vi "Methods to Method Info.vi"(10 "Class":string, 11 "Methods from Node":T2(array[cluster])) -> (2 "Methods for Tree":T1(array[cluster]), 3 "Methods[]":T3(array[cluster]))   [LabVIEW 2023] (continued)
From Typedefs"}, "Method Flags"={"IsDeprecated"=FALSE, "IsPrivate"=FALSE, "IsScripting"=FALSE, "IsNotInRun-Time"=FALSE}, "Divider"=FALSE}, {"Class Info"={"Unique ID string"="82", "Parent ID string"="", "Class Name (unlocalized)"="TagSet", "Class Name (localized)"="TagSet"}, "Method Info"={"Unique ID string"="5d1e4400", "Data name"="Get", "Short name (localized)"="Get", "Long name (localized)"="Get"}, "Method Flags"={"IsDeprecated"=FALSE, "IsPrivate"=TRUE, "IsScripting"=FALSE, "IsNotInRun-Time"=TRUE}, "Divider"=FALSE}, {"Class Info"={"Unique ID string"="82", "Parent ID string"="", "Class Name (unlocalized)"="TagSet", "Class Name (localized)"="TagSet"}, "Method Info"={"Unique ID string"="5d1e4401", "Data name"="Set", "Short name (localized)"="Set", "Long name (localized)"="Set"}, "Method Flags"={"IsDeprecated"=FALSE, "IsPrivate"=TRUE, "IsScripting"=FALSE, "IsNotInRun-Time"=TRUE}, "Divider"=FALSE}, {"Class Info"={"Unique ID string"="82", "Parent ID string"="", "Class Name (unlocalized)"="TagSet", "Class Name (localized)"="TagSet"}, "Method Info"={"Unique ID string"="5d1e4402", "Data name"="Set XML", "Short name (localized)"="Set XML", "Long name (localized)"="Set XML"}, "Method Flags"={"IsDeprecated"=FALSE, "IsPrivate"=TRUE, "IsScripting"=FALSE, "IsNotInRun-Time"=TRUE}, "Divider"=FALSE}, {"Class Info"={"Unique ID string"="82", "Parent ID string"="", "Class Name (unlocalized)"="TagSet", "Class Name (localized)"="TagSet"}, "Method Info"={"Unique ID string"="5d1e4403", "Data name"="Get XML", "Short name (localized)"="Get XML", "Long name (localized)"="Get XML"}, "Method Flags"={"IsDeprecated"=FALSE, "IsPrivate"=TRUE, "IsScripting"=FALSE, "IsNotInRun-Time"=TRUE}, "Divider"=FALSE}, {"Class Info"={"Unique ID string"="84", "Parent ID string"="123", "Class Name (unlocalized)"="SceneWindow", "Class Name (localized)"="SceneWindow"}, "Method Info"={"Unique ID string"="c55e400", "Data name"="Setup Camera", "Short name (localized)"="Setup Camera", "Long name (localized)"="Setup Camera"}, "Method Flags"={"IsDeprecated"=FALSE, "IsPrivate"=FALSE, "IsScripting"=FALSE, "IsNotInRun-Time"=FALSE}, "Divider"=FALSE}, {"Class Info"={"Unique ID string"="84", "Parent ID string"="123", "Class Name (unlocalized)"="SceneWindow", "Class Name (localized)"="SceneWindow"}, "Method Info"={"Unique ID string"="c55e401", "Data name"="Projection.Frustum", "Short name (localized)"="Projection.Frustum", "Long name (localized)"="Projection:Frustum"}, "Method Flags"={"IsDeprecated"=FALSE, "IsPrivate"=FALSE, "IsScripting"=FALSE, "IsNotInRun-Time"=FALSE}, "Divider"=FALSE}, {"Class Info"={"Unique ID string"="84", "Parent ID string"="123", "Class Name (unlocalized)"="SceneWindow", "Class Name (localized)"="SceneWindow"}, "Method Info"={"Unique ID string"="c55e402", "Data name"="Projection.Orthographic", "Short name (localized)"="Projection.Orthographic", "Long name (localized)"="Projection:Orthographic"}, "Method Flags"={"IsDeprecated"=FALSE, "IsPrivate"=FALSE, "IsScripting"=FALSE, "IsNotInRun-Time"=FALSE}, "Divider"=FALSE}, {"Class Info"={"Unique ID string"="84", "Parent ID string"="123", "Class Name (unlocalized)"="SceneWindow", "Class Name (localized)"="SceneWindow"}, "Method Info"={"Unique ID string"="c55e403", "Data name"="Projection.Perspective", "Short name (localized)"="Projection.Perspective", "Long name (localized)"="Projection:Perspective"}, "Method Flags"={"IsDeprecated"=FALSE, "IsPrivate"=FALSE, "IsScripting"=FALSE, "IsNotInRun-Time"=FALSE}, "Divider"=FALSE}, {"Class Info"={"Unique ID string"="84", "Parent ID string"="123", "Class Name (unlocalized)"="SceneWindow", "Class Name (localized)"="SceneWindow"}, "Method Info"={"Unique ID string"="c55e404", "Data name"="Render to Image", "Short name (localized)"="Render to Image", "Long name (localized)"="Render to Image"}, "Method Flags"={"IsDeprecated"=FALSE, "IsPrivate"=FALSE, "IsScripting"=FALSE, "IsNotInRun-Time"=FALSE}, "Divider"=FALSE}, {"Class Info"={"Unique ID string"="84", "Parent ID string"="123", "Class Name (unlocalized)"="SceneWindow", "Class Name (localized)"="SceneWindow"}, "Method Info"={"Unique ID string"="c55e405", "Data name"="Pick", "Short name (localized)"="Pick", "Long name (localized)"="Pick"}, "Method Flags"={"IsDeprecated"=FALSE, "IsPrivate"=FALSE, "IsScripting"=FALSE, "IsNotInRun-Time"=FALSE}, "Divider"=FALSE}, {"Class Info"={"Unique ID string"="84", "Parent ID string"="123", "Class Name (unlocalized)"="SceneWindow", "Class Name (localized)"="SceneWindow"}, "Method Info"={"Unique ID string"="c55e406", "Data name"="Redraw", "Short name (localized)"="Redraw", "Long name (localized)"="Redraw"}, "Method Flags"={"IsDeprecated"=FALSE, "IsPrivate"=FALSE, "IsScripting"=FALSE, "IsNotInRun-Time"=FALSE}, "Divider"=FALSE}, {"Class Info"={"Unique ID string"="84", "Parent ID string"="123", "Class Name (unlocalized)"="SceneWindow", "Class Name (localized)"="SceneWindow"}, "Method Info"={"Unique ID string"="c55e407", "Data name"="AutoFocus", "Short name (localized)"="AutoFocus", "Long name (localized)"="AutoFocus"}, "Method Flags"={"IsDeprecated"=FALSE, "IsPrivate"=FALSE, "IsScripting"=FALSE, "IsNotInRun-Time"=FALSE}, "Divider"=FALSE}, {"Class Info"={"Unique ID string"="84", "Parent ID string"="123", "Class Name (unlocalized)"="SceneWindow", "Class Name (localized)"="SceneWindow"}, "Method Info"={"Unique ID string"="c55e408", "Data name"="WindowToObjectCoords", "Short name (localized)"="WindowToObjectCoords", "Long name (localized)"="WindowToObjectCoords"}, "Method Flags"={"IsDeprecated"=FALSE, "IsPrivate"=FALSE, "IsScripting"=FALSE, "IsNotInRun-Time"=FALSE}, "Divider"=FALSE}, {"Class Info"={"Unique ID string"="85", "Parent ID string"="80", "Class Name (unlocalized)"="LVClassLibrary", "Class Name (localized)"="LVClassLibrary"}, "Method Info"={"Unique ID string"="97d6c01", "Data name"="Add Property", "Short name (localized)"="Add Property", "Long name (localized)"="Add Property"}, "Method Flags"={"IsDeprecated"=FALSE, "IsPrivate"=TRUE, "IsScripting"=TRUE, "IsNotInRun-Time"=FALSE}, "Divider"=FALSE}, {"Class Info"={"Unique ID string"="85", "Parent ID string"="80", "Class Name (unlocalized)"="LVClassLibrary", "Class Name (localized)"="LVClassLibrary"}, "Method Info"={"Unique ID string"="97d6c02", "Data name"="Add Dynamic Member VI", "Short name (localized)"="Add Dynamic Member VI", "Long name (localized)"="Add Dynamic Member VI"}, "Method Flags"={"IsDeprecated"=FALSE, "IsPrivate"=TRUE, "IsScripting"=TRUE, "IsNotInRun-Time"=FALSE}, "Divider"=FALSE}, {"Class Info"={"Unique ID string"="85", "Parent ID string"="80", "Class Name (unlocalized)"="LVClassLibrary", "Class Name (localized)"="LVClassLibrary"}, "Method Info"={"Unique ID string"="97d6c03", "Data name"="Add Static Member VI", "Short name (localized)"="Add Static Member VI", "Long name (localized)"="Add Static Member VI"}, "Method Flags"={"IsDeprecated"=FALSE, "IsPrivate"=TRUE, "IsScripting"=TRUE, "IsNotInRun-Time"=FALSE}, "Divider"=FALSE}, {"Class Info"={"Unique ID string"="85", "Parent ID string"="80", "Class Name (unlocalized)"="LVClassLibrary", "Class Name (localized)"="LVClassLibrary"}, "Method Info"={"Unique ID string"="97d6c04", "Data name"="Add Probe", "Short name (localized)"="Add Probe", "Long name (localized)"="Add Probe"}, "Method Flags"={"IsDeprecated"=FALSE, "IsPrivate"=TRUE, "IsScripting"=TRUE, "IsNotInRun-Time"=FALSE}, "Divider"=FALSE}, {"Class Info"={"Unique ID string"="85", "Parent ID string"="80", "Class Name (unlocalized)"="LVClassLibrary", "Class Name (localized)"="LVClassLibrary"}, "Method Info"={"Unique ID string"="97d6c05", "Data name"="Remove Property", "Short name (localized)"="Remove Property", "Long name (localized)"="Remove Property"}, "Method Flags"={"IsDeprecated"=FALSE, "IsPrivate"=TRUE, "IsScripting"=TRUE, "IsNotInRun-Time"=FALSE}, "Divider"=FALSE}, {"Class Info"={"Unique ID string"="85", "Parent ID string"="80", "Class Name (unlocalized)"="LVClassLibrary", "Class Name (localized)"="LVClassLibrary"}, "Method Info"={"Unique ID string"="97d6c06", "Data name"="Remove Member VI", "Short name (localized)"="Remove Member VI", "Long name (localized)"="Remove Member VI"}, "Method Flags"={"IsDeprecated"=FALSE, "IsPrivate"=TRUE, "IsScripting"=TRUE, "IsNotInRun-Time"=FALSE}, "Divider"=FALSE}, {"Class Info"={"Unique ID string"="85", "Parent ID string"="80", "Class Name (unlocalized)"="LVClassLibrary", "Class Name (localized)"="LVClassLibrary"}, "Method Info"={"Unique ID string"="97d6c07", "Data name"="Remove Probe", "Short name (localized)"="Remove Probe", "Long name (localized)"="Remove Probe"}, "Method Flags"={"IsDeprecated"=FALSE, "IsPrivate"=TRUE, "IsScripting"=TRUE, "IsNotInRun-Time"=FALSE}, "Divider"=FALSE}, {"Class Info"={"Unique ID string"="85", "Parent ID string"="80", "Class Name (unlocalized)"="LVClassLibrary", "Class Name (localized)"="LVClassLibrary"}, "Method Info"={"Unique ID string"="97d6c09", "Data name"="Clone Member Data", "Short name (localized)"="Clone Member Data", "Long name (localized)"="Clone Member Data"}, "Method Flags"={"IsDeprecated"=FALSE, "IsPrivate"=TRUE, "IsScripting"=TRUE, "IsNotInRun-Time"=FALSE}, "Divider"=FALSE}, {"Class Info"={"Unique ID string"="85", "Parent ID string"="80", "Class Name (unlocalized)"="LVClassLibrary", "Class Name (localized)"="LVClassLibrary"}, "Method Info"={"Unique ID string"="97d6c0a", "Data name"="Set Member Data", "Short name (localized)"="Set Member Data", "Long name (localized)"="Set Member Data"}, "Method Flags"={"IsDeprecated"=FALSE, "IsPrivate"=TRUE, "IsScripting"=TRUE, "IsNotInRun-Time"=FALSE}, "Divider"=FALSE}, {"Class Info"={"Unique ID string"="85", "Parent ID string"="80", "Class Name (unlocalized)"="LVClassLibrary", "Class Name (localized)"="LVClassLibrary"}, "Method Info"={"Unique ID string"="97d6c0b", "Data name"="Get MustOverride?", "Short name (localized)"="Get MustOverride?", "Long name (localized)"="Descendants Must Override Item?:Get"}, "Method Flags"={"IsDeprecated"=FALSE, "IsPrivate"=FALSE, "IsScripting"=FALSE, "IsNotInRun-Time"=TRUE}, "Divider"=FALSE}, {"Class Info"={"Unique ID string"="85", "Parent ID string"="80", "Class Name (unlocalized)"="LVClassLibrary", "Class Name (localized)"="LVClassLibrary"}, "Method Info"={"Unique ID string"="97d6c0c", "Data name"="Set MustOverride?", "Short name (localized)"="Set MustOverride?", "Long name (localized)"="Descendants Must Override Item?:Set"}, "Method Flags"={"IsDeprecated"=FALSE, "IsPrivate"=FALSE, "IsScripting"=FALSE, "IsNotInRun-Time"=TRUE}, "Divider"=FALSE}, {"Class Info"={"Unique ID string"="85", "Parent ID string"="80", "Class Name (unlocalized)"="LVClassLibrary", "Class Name (localized)"="LVClassLibrary"}, "Method Info"={"Unique ID string"="97d6c0d", "Data name"="Get MustCallParent?", "Short name (localized)"="Get MustCallParent?", "Long name (localized)"="Descendants Must Call Parent Item?:Get"}, "Method Flags"={"IsDeprecated"=FALSE, "IsPrivate"=FALSE, "IsScripting"=FALSE, "IsNotInRun-Time"=TRUE}, "Divider"=FALSE}, {"Class Info"={"Unique ID string"="85", "Parent ID string"="80", "Class Name (unlocalized)"="LVClassLibrary", "Class Name (localized)"="LVClassLibrary"}, "Method Info"={"Unique ID string"="97d6c0e", "Data name"="Set MustCallParent?", "Short name (localized)"="Set MustCallParent?", "Long name (localized)"="Descendants Must Call Parent Item?:Set"}, "Method Flags"={"IsDeprecated"=FALSE, "IsPrivate"=FALSE, "IsScripting"=FALSE, "IsNotInRun-Time"=TRUE}, "Divider"=FALSE}, {"Class Info"={"Unique ID string"="85", "Parent ID string"="80", "Class Name (unlocalized)"="LVClassLibrary", "Class Name (localized)"="LVClassLibrary"}, "Method Info"={"Unique ID string"="97d6c0f", "Data name"="HasImplementation", "Short name (localized)"="HasImplementation", "Long name (localized)"="Has Implementation?"}, "Method Flags"={"IsDeprecated"=FALSE, "IsPrivate"=FALSE, "IsScripting"=FALSE, "IsNotInRun-Time"=TRUE}, "Divider"=FALSE}, {"Class Info"={"Unique ID string"="85", "Parent ID string"="80", "Class Name (unlocalized)"="LVClassLibrary", "Class Name (localized)"="LVClassLibrary"}, "Method Info"={"Unique ID string"="97d6c10", "Data name"="Get Prop Def Folder by Unique ID", "Short name (localized)"="Get Prop Def Folder by Unique ID", "Long name (localized)"="Get Property Definition Folder by Unique ID"}, "Method Flags"={"IsDeprecated"=FALSE, "IsPrivate"=TRUE, "IsScripting"=TRUE, "IsNotInRun-Time"=TRUE}, "Divider"=FALSE}, {"Class Info"={"Unique ID string"="85", "Parent ID string"="80", "Class Name (unlocalized)"="LVClassLibrary", "Class Name (localized)"="LVClassLibrary"}, "Method Info"={"Unique ID string"="97d6c11", "Data name"="DeParent Class", "Short name (localized)"="DeParent Class", "Long name (localized)"="DeParent Class"}, "Method Flags"={"IsDeprecated"=FALSE, "IsPrivate"=TRUE, "IsScripting"=TRUE, "IsNotInRun-Time"=TRUE}, "Divider"=FALSE}, {"Class Info"={"Unique ID string"="87", "Parent ID string"="2", "Class Name (unlocalized)"="MethodVI", "Class Name (localized)"="MethodVI"}, "Method Info"={"Unique ID string"="69a73c00", "Data name"="Invoke Method Editor", "Short name (localized)"="Invoke Method Editor", "Long name (localized)"="Invoke Method Editor"}, "Method Flags"={"IsDeprecated"=FALSE, "IsPrivate"=TRUE, "IsScripting"=FALSE, "IsNotInRun-Time"=FALSE}, "Divider"=FALSE}, {"Class Info"={"Unique ID string"="91", "Parent ID string"="", "Class Name (unlocalized)"="LVTarget", "Class Name (localized)"="LVTarget"}, "Method Info"={"Unique ID string"="5d37bc00", "Data name"="Get Attributes", "Short name (localized)"="Get Attributes", "Long name (localized)"="Get Attributes"}, "Method Flags"={"IsDeprecated"=FALSE, "IsPrivate"=TRUE, "IsScripting"=FALSE, "IsNotInRun-Time"=FALSE}, "Divider"=FALSE}, {"Class Info"={"Unique ID string"="91", "Parent ID string"="", "Class Name (unlocalized)"="LVTarget", "Class Name (localized)"="LVTarget"}, "Method Info"={"Unique ID string"="5d37bc01", "Data name"="Set Attributes", "Short name (localized)"="Set Attributes", "Long name (localized)"="Set Attributes"}, "Method Flags"={"IsDeprecated"=FALSE, "IsPrivate"=TRUE, "IsScripting"=FALSE, "IsNotInRun-Time"=FALSE}, "Divider"=FALSE}, {"Class Info"={"Unique ID string"="91", "Parent ID string"="", "Class Name (unlocalized)"="LVTarget", "Class Name (localized)"="LVTarget"}, "Method Info"={"Unique ID string"="5d37bc02", "Data name"="Custom Command", "Short name (localized)"="Custom Command", "Long name (localized)"="Custom Command"}, "Method Flags"={"IsDeprecated"=FALSE, "IsPrivate"=TRUE, "IsScripting"=FALSE, "IsNotInRun-Time"=FALSE}, "Divider"=FALSE}, {"Class Info"={"Unique ID string"="91", "Parent ID string"="", "Class Name (unlocalized)"="LVTarget", "Class Name (localized)"="LVTarget"}, "Method Info"={"Unique ID string"="5d37c003", "Data name"="LocateFile", "Short name (localized)"="LocateFile", "Long name (localized)"="Locate File or Folder"}, "Method Flags"={"IsDeprecated"=FALSE, "IsPrivate"=TRUE, "IsScripting"=FALSE, "IsNotInRun-Time"=FALSE}, "Divider"=FALSE}, {"Class Info"={"Unique ID string"="91", "Parent ID string"="", "Class Name (unlocalized)"="LVTarget", "Class Name (localized)"="LVTarget"}, "Method Info"={"Unique ID string"="5d37c004", "Data name"="DirChain", "Short name (localized)"="DirChain", "Long name (localized)"="Directory Chain"}, "Method Flags"={"IsDeprecated"=FALSE, "IsPrivate"=TRUE, "IsScripting"=TRUE, "IsNotInRun-Time"=FALSE}, "Divider"=FALSE}, {"Class Info"={"Unique ID string"="91", "Parent ID string"="", "Class Name (unlocalized)"="LVTarget", "Class Name (localized)"="LVTarget"}, "Method Info"={"Unique ID string"="5d37c005", "Data name"="ResolveSymbolicPaths", "Short name (localized)"="ResolveSymbolicPaths", "Long name (localized)"="Resolve Symbolic Paths"}, "Method Flags"={"IsDeprecated"=FALSE, "IsPrivate"=TRUE, "IsScripting"=FALSE, "IsNotInRun-Time"=FALSE}, "Divider"=FALSE}, {"Class Info"={"Unique ID string"="91", "Parent ID string"="", "Class Name (unlocalized)"="LVTarget", "Class Name (localized)"="LVTarget"}, "Method Info"={"Unique ID string"="5d37c006", "Data name"="ToSymbolicOrRelativePath", "Short name (localized)"="ToSymbolicOrRelativePath", "Long name (localized)"="Convert to Symbolic Or Relative Path"}, "Method Flags"={"IsDeprecated"=FALSE, "IsPrivate"=TRUE, "IsScripting"=FALSE, "IsNotInRun-Time"=FALSE}, "Divider"=FALSE}, {"Class Info"={"Unique ID string"="91", "Parent ID string"="", "Class Name (unlocalized)"="LVTarget", "Class Name (localized)"="LVTarget"}, "Method Info"={"Unique ID string"="5d37c007", "Data name"="Update Target Syntax", "Short name (localized)"="Update Target Syntax", "Long name (localized)"="Update Target Syntax"}, "Method Flags"={"IsDeprecated"=FALSE, "IsPrivate"=TRUE, "IsScripting"=FALSE, "IsNotInRun-Time"=FALSE}, "Divider"=FALSE}, {"Class Info"={"Unique ID string"="92", "Parent ID string"="22", "Class Name (unlocalized)"="MixedSignalGraph", "Class Name (localized)"="MixedSignalGraph"}, "Method Info"={"Unique ID string"="393e8800", "Data name"="Export Image", "Short name (localized)"="Export Image", "Long name (localized)"="Export Image"}, "Method Flags"={"IsDeprecated"=FALSE, "IsPrivate"=FALSE, "IsScripting"=FALSE, "IsNotInRun-Time"=FALSE}, "Divider"=FALSE}, {"Class Info"={"Unique ID string"="92", "Parent ID string"="22", "Class Name (unlocalized)"="MixedSignalGraph", "Class Name (localized)"="MixedSignalGraph"}, "Method Info"={"Unique ID string"="393e8801", "Data name"="Export Image Color", "Short name (localized)"="Export Image Color", "Long name (localized)"="Export Image Color"}, "Method Flags"={"IsDeprecated"=FALSE, "IsPrivate"=TRUE, "IsScripting"=FALSE, "IsNotInRun-Time"=FALSE}, "Divider"=FALSE}, {"Class Info"={"Unique ID string"="92", "Parent ID string"="22", "Class Name (unlocalized)"="MixedSignalGraph", "Class Name (localized)"="MixedSignalGraph"}, "Method Info"={"Unique ID string"="393e8802", "Data name"="Export Data to Clipboard", "Short name (localized)"="Export Data to Clipboard", "Long name (localized)"="Export Data to Clipboard"}, "Method Flags"={"IsDeprecated"=FALSE, "IsPrivate"=FALSE, "IsScripting"=FALSE, "IsNotInRun-Time"=FALSE}, "Divider"=FALSE}, {"Class Info"={"Unique ID string"="92", "Parent ID string"="22", "Class Name (unlocalized)"="MixedSignalGraph", "Class Name (localized)"="MixedSignalGraph"}, "Method Info"={"Unique ID string"="393e8803", "Data name"="Export Data to Excel", "Short name (localized)"="Export Data to Excel", "Long name (localized)"="Export Data to Excel"}, "Method Flags"={"IsDeprecated"=FALSE, "IsPrivate"=FALSE, "IsScripting"=FALSE, "IsNotInRun-Time"=FALSE}, "Divider"=FALSE}, {"Class Info"={"Unique ID string"="92", "Parent ID string"="22", "Class Name (unlocalized)"="MixedSignalGraph", "Class Name (localized)"="MixedSignalGraph"}, "Method Info"={"Unique ID string"="393e8804", "Data name"="Export Data to DIAdem", "Short name (localized)"="Export Data to DIAdem", "Long name (localized)"="Export Data to DIAdem"}, "Method Flags"={"IsDeprecated"=FALSE, "IsPrivate"=FALSE, "IsScripting"=FALSE, "IsNotInRun-Time"=FALSE}, "Divider"=FALSE}, {"Class Info"={"Unique ID string"="92", "Parent ID string"="22", "Class Name (unlocalized)"="MixedSignalGraph", "Class Name (localized)"="MixedSignalGraph"}, "Method Info"={"Unique ID string"="393e8805", "Data name"="Export Plot Data To Clipboard", "Short name (localized)"="Export Plot Data To Clipboard", "Long name (localized)"="Export Plot Data To Clipboard"}, "Method Flags"={"IsDeprecated"=FALSE, "IsPrivate"=FALSE, "IsScripting"=FALSE, "IsNotInRun-Time"=FALSE}, "Divider"=FALSE}, {"Class Info"={"Unique ID string"="92", "Parent ID string"="22", "Class Name (unlocalized)"="MixedSignalGraph", "Class Name (localized)"="MixedSignalGraph"}, "Method Info"={"Unique ID string"="393e8806", "Data name"="Export Plot Data To Excel", "Short name (localized)"="Export Plot Data To Excel", "Long name (localized)"="Export Plot Data To Excel"}, "Method Flags"={"IsDeprecated"=FALSE, "IsPrivate"=FALSE, "IsScripting"=FALSE, "IsNotInRun-Time"=FALSE}, "Divider"=FALSE}, {"Class Info"={"Unique ID string"="92", "Parent ID string"="22", "Class Name (unlocalized)"="MixedSignalGraph", "Class Name (localized)"="MixedSignalGraph"}, "Method Info"={"Unique ID string"="393e8807", "Data name"="Export Plot Data To DIAdem", "Short name (localized)"="Export Plot Data To DIAdem", "Long name (localized)"="Export Plot Data To DIAdem"}, "Method Flags"={"IsDeprecated"=FALSE, "IsPrivate"=FALSE, "IsScripting"=FALSE, "IsNotInRun-Time"=FALSE}, "Divider"=FALSE}, {"Class Info"={"Unique ID string"="93", "Parent ID string"="", "Class Name (unlocalized)"="Provider", "Class Name (localized)"="Provider"}, "Method Info"={"Unique ID string"="46e29800", "Data name"="GetItemTypesForItem", "Short name (localized)"="GetItemTypesForItem", "Long name (localized)"="Get Item Types For Item"}, "Method Flags"={"IsDeprecated"=FALSE, "IsPrivate"=TRUE, "IsScripting"=FALSE, "IsNotInRun-Time"=TRUE}, "Divider"=FALSE}, {"Class Info"={"Unique ID string"="94", "Parent ID string"="", "Class Name (unlocalized)"="CopyOperation", "Class Name (localized)"="CopyOperation"}, "Method Info"={"Unique ID string"="7f2be000", "Data name"="Copy Items", "Short name (localized)"="Copy Items", "Long name (localized)"="Copy Items"}, "Method Flags"={"IsDeprecated"=FALSE, "IsPrivate"=TRUE, "IsScripting"=FALSE, "IsNotInRun-Time"=TRUE}, "Divider"=FALSE}, {"Class Info"={"Unique ID string"="94", "Parent ID string"="", "Class Name (unlocalized)"="CopyOperation", "Class Name (localized)"="CopyOperation"}, "Method Info"={"Unique ID string"="7f2be001", "Data name"="End", "Short name (localized)"="End", "Long name (localized)"="End"}, "Method Flags"={"IsDeprecated"=FALSE, "IsPrivate"=TRUE, "IsScripting"=FALSE, "IsNotInRun-Time"=TRUE}, "Divider"=FALSE}, {"Class Info"={"Unique ID string"="94", "Parent ID string"="", "Class Name (unlocalized)"="CopyOperation", "Class Name (localized)"="CopyOperation"}, "Method Info"={"Unique ID string"="7f2be002", "Data name"="MapProjectItemToCopyItem", "Short name (localized)"="MapProjectItemToCopyItem", "Long name (localized)"="Map Project Item To Copy Item"}, "Method Flags"={"IsDeprecated"=FALSE, "IsPrivate"=TRUE, "IsScripting"=FALSE, "IsNotInRun-Time"=TRUE}, "Divider"=FALSE}, {"Class Info"={"Unique ID string"="94", "Parent ID string"="", "Class Name (unlocalized)"="CopyOperation", "Class Name (localized)"="CopyOperation"}, "Method Info"={"Unique ID string"="7f2be003", "Data name"="CopyItem", "Short name (localized)"="CopyItem", "Long name (localized)"="Copy Item"}, "Method Flags"={"IsDeprecated"=FALSE, "IsPrivate"=TRUE, "IsScripting"=FALSE, "IsNotInRun-Time"=TRUE}, "Divider"=FALSE}, {"Class Info"={"Unique ID string"="94", "Parent ID string"="", "Class Name (unlocalized)"="CopyOperation", "Class Name (localized)"="CopyOperation"}, "Method Info"={"Unique ID string"="7f2be004", "Data name"="Begin", "Short name (localized)"="Begin", "Long name (localized)"="Begin"}, "Method Flags"={"IsDeprecated"=FALSE, "IsPrivate"=TRUE, "IsScripting"=FALSE, "IsNotInRun-Time"=TRUE}, "Divider"=FALSE}, {"Class Info"={"Unique ID string"="94", "Parent ID string"="", "Class Name (unlocalized)"="CopyOperation", "Class Name (localized)"="CopyOperation"}, "Method Info"={"Unique ID string"="7f2be005", "Data name"="Peek", "Short name (localized)"="Peek", "Long name (localized)"="Peek"}, "Method Flags"={"IsDeprecated"=FALSE, "IsPrivate"=TRUE, "IsScripting"=FALSE, "IsNotInRun-Time"=TRUE}, "Divider"=FALSE}, {"Class Info"={"Unique ID string"="94", "Parent ID string"="", "Class Name (unlocalized)"="CopyOperation", "Class Name (localized)"="CopyOperation"}, "Method Info"={"Unique ID string"="7f2be006", "Data name"="Next", "Short name (localized)"="Next", "Long name (localized)"="Next"}, "Method Flags"={"IsDeprecated"=FALSE, "IsPrivate"=TRUE, "IsScripting"=FALSE, "IsNotInRun-Time"=TRUE}, "Divider"=FALSE}, {"Class Info"={"Unique ID string"="94", "Parent ID string"="", "Class Name (unlocalized)"="CopyOperation", "Class Name (localized)"="CopyOperation"}, "Method Info"={"Unique ID string"="7f2be007", "Data name"="Find Item", "Short name (localized)"="Find Item", "Long name (localized)"="Find Item"}, "Method Flags"={"IsDeprecated"=FALSE, "IsPrivate"=TRUE, "IsScripting"=FALSE, "IsNotInRun-Time"=TRUE}, "Divider"=FALSE}, {"Class Info"={"Unique ID string"="95", "Parent ID string"="74", "Class Name (unlocalized)"="TargetItem", "Class Name (localized)"="TargetItem"}, "Method Info"={"Unique ID string"="6851e400", "Data name"="Refresh Dependencies", "Short name (localized)"="Refresh Dependencies", "Long name (localized)"="Refresh Dependencies"}, "Method Flags"={"IsDeprecated"=FALSE, "IsPrivate"=FALSE, "IsScripting"=FALSE, "IsNotInRun-Time"=TRUE}, "Divider"=FALSE}, {"Class Info"={"Unique ID string"="95", "Parent ID string"="74", "Class Name (unlocalized)"="TargetItem", "Class Name (localized)"="TargetItem"}, "Method Info"={"Unique ID string"="6851e401", "Data name"="Refresh Dependencies Copy", "Short name (localized)"="Refresh Dependencies Copy", "Long name (localized)"="Refresh Dependencies Copy"}, "Method Flags"={"IsDeprecated"=FALSE, "IsPrivate"=TRUE, "IsScripting"=FALSE, "IsNotInRun-Time"=TRUE}, "Divider"=FALSE}, {"Class Info"={"Unique ID string"="95", "Parent ID string"="74", "Class Name (unlocalized)"="TargetItem", "Class Name (localized)"="TargetItem"}, "Method Info"={"Unique ID string"="6851e402", "Data name"="Refresh Dependencies Shallow", "Short name (localized)"="Refresh Dependencies Shallow", "Long name (localized)"="Refresh Dependencies Shallow"}, "Method Flags"={"IsDeprecated"=FALSE, "IsPrivate"=TRUE, "IsScripting"=FALSE, "IsNotInRun-Time"=TRUE}, "Divider"=FALSE}, {"Class Info"={"Unique ID string"="95", "Parent ID string"="74", "Class Name (unlocalized)"="TargetItem", "Class Name (localized)"="TargetItem"}, "Method Info"={"Unique ID string"="6851e403", "Data name"="GetProjectItemRefForFile", "Short name (localized)"="GetProjectItemRefForFile", "Long name (localized)"="Get ProjectItemRef For File"}, "Method Flags"={"IsDeprecated"=FALSE, "IsPrivate"=TRUE, "IsScripting"=FALSE, "IsNotInRun-Time"=FALSE}, "Divider"=FALSE}, {"Class Info"={"Unique ID string"="96", "Parent ID string"="", "Class Name (unlocalized)"="ProjectItemType", "Class Name (localized)"="ProjectItemType"}, "Method Info"={"Unique ID string"="2707f000", "Data name"="CreateInstance", "Short name (localized)"="CreateInstance", "Long name (localized)"="Create Instance"}, "Method Flags"={"IsDeprecated"=FALSE, "IsPrivate"=TRUE, "IsScripting"=FALSE, "IsNotInRun-Time"=TRUE}, "Divider"=FALSE}, {"Class Info"={"Unique ID string"="98", "Parent ID string"="", "Class Name (unlocalized)"="CopyConflict", "Class Name (localized)"="CopyConflict"}, "Method Info"={"Unique ID string"="38d7fc00", "Data name"="CompleteRefresh", "Short name (localized)"="CompleteRefresh", "Long name (localized)"="Complete Refresh"}, "Method Flags"={"IsDeprecated"=FALSE, "IsPrivate"=TRUE, "IsScripting"=FALSE, "IsNotInRun-Time"=TRUE}, "Divider"=FALSE}, {"Class Info"={"Unique ID string"="100", "Parent ID string"="6", "Class Name (unlocalized)"="SceneGraphDisplay", "Class Name (localized)"="SceneGraphDisplay"}, "Method Info"={"Unique ID string"="50f27000", "Data name"="Setup Camera", "Short name (localized)"="Setup Camera", "Long name (localized)"="Setup Camera"}, "Method Flags"={"IsDeprecated"=FALSE, "IsPrivate"=FALSE, "IsScripting"=FALSE, "IsNotInRun-Time"=FALSE}, "Divider"=FALSE}, {"Class Info"={"Unique ID string"="100", "Parent ID string"="6", "Class Name (unlocalized)"="SceneGraphDisplay", "Class Name (localized)"="SceneGraphDisplay"}, "Method Info"={"Unique ID string"="50f27002", "Data name"="Projection.Orthographic", "Short name (localized)"="Projection.Orthographic", "Long name (localized)"="Projection:Orthographic"}, "Method Flags"={"IsDeprecated"=FALSE, "IsPrivate"=FALSE, "IsScripting"=FALSE, "IsNotInRun-Time"=FALSE}, "Divider"=FALSE}, {"Class Info"={"Unique ID string"="100", "Parent ID string"="6", "Class Name (unlocalized)"="SceneGraphDisplay", "Class Name (localized)"="SceneGraphDisplay"}, "Method Info"={"Unique ID string"="50f27003", "Data name"="Projection.Perspective", "Short name (localized)"="Projection.Perspective", "Long name (localized)"="Projection:Perspective"}, "Method Flags"={"IsDeprecated"=FALSE, "IsPrivate"=FALSE, "IsScripting"=FALSE, "IsNotInRun-Time"=FALSE}, "Divider"=FALSE}, {"Class Info"={"Unique ID string"="100", "Parent ID string"="6", "Class Name (unlocalized)"="SceneGraphDisplay", "Class Name (localized)"="SceneGraphDisplay"}, "Method Info"={"Unique ID string"="50f27004", "Data name"="Render to Image", "Short name (localized)"="Render to Image", "Long name (localized)"="Render to Image"}, "Method Flags"={"IsDeprecated"=FALSE, "IsPrivate"=FALSE, "IsScripting"=FALSE, "IsNotInRun-Time"=FALSE}, "Divider"=FALSE}, {"Class Info"={"Unique ID string"="100", "Parent ID string"="6", "Class Name (unlocalized)"="SceneGraphDisplay", "Class Name (localized)"="SceneGraphDisplay"}, "Method Info"={"Unique ID string"="50f27005", "Data name"="Projection.Frustum", "Short name (localized)"="Projection.Frustum", "Long name (localized)"="Projection:Frustum"}, "Method Flags"={"IsDeprecated"=FALSE, "IsPrivate"=FALSE, "IsScripting"=FALSE, "IsNotInRun-Time"=FALSE}, "Divider"=FALSE}, {"Class Info"={"Unique ID string"="100", "Parent ID string"="6", "Class Name (unlocalized)"="SceneGraphDisplay", "Class Name (localized)"="SceneGraphDisplay"}, "Method Info"={"Unique ID string"="50f27006", "Data name"="Pick Model", "Short name (localized)"="Pick Model", "Long name (localized)"="Pick Model"}, "Method Flags"={"IsDeprecated"=FALSE, "IsPrivate"=FALSE, "IsScripting"=FALSE, "IsNotInRun-Time"=FALSE}, "Divider"=FALSE}, {"Class Info"={"Unique ID string"="100", "Parent ID string"="6", "Class Name (unlocalized)"="SceneGraphDisplay", "Class Name (localized)"="SceneGraphDisplay"}, "Method Info"={"Unique ID string"="50f27007", "Data name"="Redraw", "Short name (localized)"="Redraw", "Long name (localized)"="Redraw"}, "Method Flags"={"IsDeprecated"=FALSE, "IsPrivate"=FALSE, "IsScripting"=FALSE, "IsNotInRun-Time"=FALSE}, "Divider"=FALSE}, {"Class Info"={"Unique ID string"="100", "Parent ID string"="6", "Class Name (unlocalized)"="SceneGraphDisplay", "Class Name (localized)"="SceneGraphDisplay"}, "Method Info"={"Unique ID string"="50f27008", "Data name"="PickPoint", "Short name (localized)"="PickPoint", "Long name (localized)"="PickPoint"}, "Method Flags"={"IsDeprecated"=FALSE, "IsPrivate"=FALSE, "IsScripting"=FALSE, "IsNotInRun-Time"=FALSE}, "Divider"=FALSE}, {"Class Info"={"Unique ID string"="100", "Parent ID string"="6", "Class Name (unlocalized)"="SceneGraphDisplay", "Class Name (localized)"="SceneGraphDisplay"}, "Method Info"={"Unique ID string"="50f27009", "Data name"="AutoFocus", "Short name (localized)"="AutoFocus", "Long name (localized)"="AutoFocus"}, "Method Flags"={"IsDeprecated"=FALSE, "IsPrivate"=FALSE, "IsScripting"=FALSE, "IsNotInRun-Time"=FALSE}, "Divider"=FALSE}, {"Class Info"={"Unique ID string"="100", "Parent ID string"="6", "Class Name (unlocalized)"="SceneGraphDisplay", "Class Name (localized)"="SceneGraphDisplay"}, "Method Info"={"Unique ID string"="50f2700a", "Data name"="WindowToObjectCoords", "Short name (localized)"="WindowToObjectCoords", "Long name (localized)"="WindowToObjectCoords"}, "Method Flags"={"IsDeprecated"=FALSE, "IsPrivate"=FALSE, "IsScripting"=FALSE, "IsNotInRun-Time"=FALSE}, "Divider"=FALSE}, {"Class Info"={"Unique ID string"="101", "Parent ID string"="2", "Class Name (unlocalized)"="PolymorphicVI", "Class Name (localized)"="PolymorphicVI"}, "Method Info"={"Unique ID string"="211c2c00", "Data name"="GetPolyCHImage", "Short name (localized)"="GetPolyCHImage", "Long name (localized)"="GetPolyCHImage"}, "Method Flags"={"IsDeprecated"=FALSE, "IsPrivate"=FALSE, "IsScripting"=TRUE, "IsNotInRun-Time"=TRUE}, "Divider"=FALSE}, {"Class Info"={"Unique ID string"="102", "Parent ID string"="6", "Class Name (unlocalized)"="LabVIEWClassControl", "Class Name (localized)"="LabVIEWClassControl"}, "Method Info"={"Unique ID string"="250f9800", "Data name"="ReplaceWithControlOfOtherClass", "Short name (localized)"="ReplaceWithControlOfOtherClass", "Long name (localized)"="ReplaceWithControlOfOtherClass"}, "Method Flags"={"IsDeprecated"=FALSE, "IsPrivate"=FALSE, "IsScripting"=TRUE, "IsNotInRun-Time"=TRUE}, "Divider"=FALSE}, {"Class Info"={"Unique ID string"="103", "Parent ID string"="80", "Class Name (unlocalized)"="XInterfaceLibrary", "Class Name (localized)"="XInterfaceLibrary"}, "Method Info"={"Unique ID string"="6f2ec01", "Data name"="Add Ability", "Short name (localized)"="Add Ability", "Long name (localized)"="Add Ability"}, "Method Flags"={"IsDeprecated"=FALSE, "IsPrivate"=FALSE, "IsScripting"=FALSE, "IsNotInRun-Time"=TRUE}, "Divider"=FALSE}, {"Class Info"={"Unique ID string"="103", "Parent ID string"="80", "Class Name (unlocalized)"="XInterfaceLibrary", "Class Name (localized)"="XInterfaceLibrary"}, "Method Info"={"Unique ID string"="6f2ec03", "Data name"="Add Method", "Short name (localized)"="Add Method", "Long name (localized)"="Add Method"}, "Method Flags"={"IsDeprecated"=FALSE, "IsPrivate"=FALSE, "IsScripting"=FALSE, "IsNotInRun-Time"=TRUE}, "Divider"=FALSE}, {"Class Info"={"Unique ID string"="103", "Parent ID string"="80", "Class Name (unlocalized)"="XInterfaceLibrary", "Class Name (localized)"="XInterfaceLibrary"}, "Method Info"={"Unique ID string"="6f2ec04", "Data name"="New Prop", "Short name (localized)"="New Prop", "Long name (localized)"="New Property"}, "Method Flags"={"IsDeprecated"=FALSE, "IsPrivate"=FALSE, "IsScripting"=FALSE, "IsNotInRun-Time"=TRUE}, "Divider"=FALSE}, {"Class Info"={"Unique ID string"="103", "Parent ID string"="80", "Class Name (unlocalized)"="XInterfaceLibrary", "Class Name (localized)"="XInterfaceLibrary"}, "Method Info"={"Unique ID string"="6f2ec05", "Data name"="Unlock For Edit", "Short name (localized)"="Unlock For Edit", "Long name (localized)"="Unlock For Edit"}, "Method Flags"={"IsDeprecated"=FALSE, "IsPrivate"=TRUE, "IsScripting"=FALSE, "IsNotInRun-Time"=TRUE}, "Divider"=FALSE}, {"Class Info"={"Unique ID string"="103", "Parent ID string"="80", "Class Name (unlocalized)"="XInterfaceLibrary", "Class Name (localized)"="XInterfaceLibrary"}, "Method Info"={"Unique ID string"="6f2ec06", "Data name"="Apply Changes To Instances", "Short name (localized)"="Apply Changes To Instances", "Long name (localized)"="Apply Changes To Instances"}, "Method Flags"={"IsDeprecated"=FALSE, "IsPrivate"=TRUE, "IsScripting"=FALSE, "IsNotInRun-Time"=TRUE}, "Divider"=FALSE}, {"Class Info"={"Unique ID string"="103", "Parent ID string"="80", "Class Name (unlocalized)"="XInterfaceLibrary", "Class Name (localized)"="XInterfaceLibrary"}, "Method Info"={"Unique ID string"="6f2ec07", "Data name"="GetHelpInfo", "Short name (localized)"="GetHelpInfo", "Long name (localized)"="Get Palette Help Information"}, "Method Flags"={"IsDeprecated"=FALSE, "IsPrivate"=TRUE, "IsScripting"=FALSE, "IsNotInRun-Time"=FALSE}, "Divider"=FALSE}, {"Class Info"={"Unique ID string"="105", "Parent ID string"="104", "Class Name (unlocalized)"="SceneObject", "Class Name (localized)"="SceneObject"}, "Method Info"={"Unique ID string"="2d877400", "Data name"="Object.Add Object", "Short name (localized)"="Object.Add Object", "Long name (localized)"="Object:Add Object"}, "Method Flags"={"IsDeprecated"=FALSE, "IsPrivate"=FALSE, "IsScripting"=FALSE, "IsNotInRun-Time"=FALSE}, "Divider"=FALSE}, {"Class Info"={"Unique ID string"="105", "Parent ID string"="104", "Class Name (unlocalized)"="SceneObject", "Class Name (localized)"="SceneObject"}, "Method Info"={"Unique ID string"="2d877409", "Data name"="Object.Object Count", "Short name (localized)"="Object.Object Count", "Long name (localized)"="Object:Object Count"}, "Method Flags"={"IsDeprecated"=FALSE, "IsPrivate"=FALSE, "IsScripting"=FALSE, "IsNotInRun-Time"=FALSE}, "Divider"=FALSE}, {"Class Info"={"Unique ID string"="105", "Parent ID string"="104", "Class Name (unlocalized)"="SceneObject", "Class Name (localized)"="SceneObject"}, "Method Info"={"Unique ID string"="2d877415", "Data name"="Object.Remove Object", "Short name (localized)"="Object.Remove Object", "Long name (localized)"="Object:Remove Object"}, "Method Flags"={"IsDeprecated"=FALSE, "IsPrivate"=FALSE, "IsScripting"=FALSE, "IsNotInRun-Time"=FALSE}, "Divider"=FALSE}, {"Class Info"={"Unique ID string"="105", "Parent ID string"="104", "Class Name (unlocalized)"="SceneObject", "Class Name (localized)"="SceneObject"}, "Method Info"={"Unique ID string"="2d877416", "Data name"="Transformation.Rotate", "Short name (localized)"="Transformation.Rotate", "Long name (localized)"="Transformation:Rotate"}, "Method Flags"={"IsDeprecated"=FALSE, "IsPrivate"=FALSE, "IsScripting"=FALSE, "IsNotInRun-Time"=FALSE}, "Divider"=FALSE}, {"Class Info"={"Unique ID string"="105", "Parent ID string"="104", "Class Name (unlocalized)"="SceneObject", "Class Name (localized)"="SceneObject"}, "Method Info"={"Unique ID string"="2d877417", "Data name"="Transformation.Translate", "Short name (localized)"="Transformation.Translate", "Long name (localized)"="Transformation:Translate"}, "Method Flags"={"IsDeprecated"=FALSE, "IsPrivate"=FALSE, "IsScripting"=FALSE, "IsNotInRun-Time"=FALSE}, "Divider"=FALSE}, {"Class Info"={"Unique ID string"="105", "Parent ID string"="104", "Class Name (unlocalized)"="SceneObject", "Class Name (localized)"="SceneObject"}, "Method Info"={"Unique ID string"="2d877418", "Data name"="Transformation.Scale", "Short name (localized)"="Transformation.Scale", "Long name (localized)"="Transformation:Scale"}, "Method Flags"={"IsDeprecated"=FALSE, "IsPrivate"=FALSE, "IsScripting"=FALSE, "IsNotInRun-Time"=FALSE}, "Divider"=FALSE}, {"Class Info"={"Unique ID string"="105", "Parent ID string"="104", "Class Name (unlocalized)"="SceneObject", "Class Name (localized)"="SceneObject"}, "Method Info"={"Unique ID string"="2d877419", "Data name"="Transformation.Set Rotation", "Short name (localized)"="Transformation.Set Rotation", "Long name (localized)"="Transformation:Set Rotation"}, "Method Flags"={"IsDeprecated"=FALSE, "IsPrivate"=FALSE, "IsScripting"=FALSE, "IsNotInRun-Time"=FALSE}, "Divider"=FALSE}, {"Class Info"={"Unique ID string"="105", "Parent ID string"="104", "Class Name (unlocalized)"="SceneObject", "Class Name (localized)"="SceneObject"}, "Method Info"={"Unique ID string"="2d87741a", "Data name"="Transformation.SetTranslation", "Short name (localized)"="Transformation.SetTranslation", "Long name (localized)"="Transformation:Set Translation"}, "Method Flags"={"IsDeprecated"=FALSE, "IsPrivate"=FALSE, "IsScripting"=FALSE, "IsNotInRun-Time"=FALSE}, "Divider"=FALSE}, {"Class Info"={"Unique ID string"="105", "Parent ID string"="104", "Class Name (unlocalized)"="SceneObject", "Class Name (localized)"="SceneObject"}, "Method Info"={"Unique ID string"="2d87741b", "Data name"="Transformation.Set Scale", "Short name (localized)"="Transformation.Set Scale", "Long name (localized)"="Transformation:Set Scale"}, "Method Flags"={"IsDeprecated"=FALSE, "IsPrivate"=FALSE, "IsScripting"=FALSE, "IsNotInRun-Time"=FALSE}, "Divider"=FALSE}, {"Class Info"={"Unique ID string"="105", "Parent ID string"="104", "Class Name (unlocalized)"="SceneObject", "Class Name (localized)"="SceneObject"}, "Method Info"={"Unique ID string"="2d87741c", "Data name"="Transformation.Clear", "Short name (localized)"="Transformation.Clear", "Long name (localized)"="Transformation:Clear"}, "Method Flags"={"IsDeprecated"=FALSE, "IsPrivate"=FALSE, "IsScripting"=FALSE, "IsNotInRun-Time"=FALSE}, "Divider"=FALSE}, {"Class Info"={"Unique ID string"="105", "Parent ID string"="104", "Class Name (unlocalized)"="SceneObject", "Class Name (localized)"="SceneObject"}, "Method Info"={"Unique ID string"="2d87741d", "Data name"="Light.Get State", "Short name (localized)"="Light.Get State", "Long name (localized)"="Light:Get State"}, "Method Flags"={"IsDeprecated"=FALSE, "IsPrivate"=FALSE, "IsScripting"=FALSE, "IsNotInRun-Time"=FALSE}, "Divider"=FALSE}, {"Class Info"={"Unique ID string"="105", 
